vi "CANOpen_SDO Read RW.vi"(8 "error in":errorcluster, 11 "SDO Asynch in":T1 {"HW Dyn Read"."Resp Chan."."Chan Refs" format="%.0x"; "HW Dyn Read"."Req Chan."."Chan Refs" format="%.0x"; "HW Dyn Write"."Resp Chan."."Chan Refs" format="%.0x"; "HW Dyn Write"."Req Chan."."Chan Refs" format="%.0x"; "List SDO"."Resp Chan."."Chan Refs" format="%.0x"; "List SDO"."Req Chan."."Chan Refs" format="%.0x"}) -> (0 "error out":errorcluster, 3 "SDO Asynch out":T1 {"HW Dyn Read"."Resp Chan."."Chan Refs" format="%.0x"; "HW Dyn Read"."Req Chan."."Chan Refs" format="%.0x"; "HW Dyn Write"."Resp Chan."."Chan Refs" format="%.0x"; "HW Dyn Write"."Req Chan."."Chan Refs" format="%.0x"; "List SDO"."Resp Chan."."Chan Refs" format="%.0x"; "List SDO"."Req Chan."."Chan Refs" format="%.0x"})   [LabVIEW 2021, in "CANOpen Addon Engine.lvlib"]
uses:
  CANOpen Addon Engine.lvlib
  CANOpen_VS SDOs Data Refs.ctl
  <vilib>/NI VeriStand/Custom Device API/Data Reference.ctl
  Async VIs/CANOpen_Main/SubVIs/CanOpen_SDO Dynamic queue.ctl
  Shared/CANOpen_SDO queue W data.ctl
  Shared/CANOpen_SDO queue mode.ctl
  Shared/CANOpen_PDO Data Type in queue.ctl
  <vilib>/NI VeriStand/Custom Device API/Global Data Refs.vi
  <vilib>/NI VeriStand/Custom Device API/Custom Device API.lvlib
  Debug/SubVIs/Global debug.vi
  Shared/CANOpen Addon Shared.lvlib
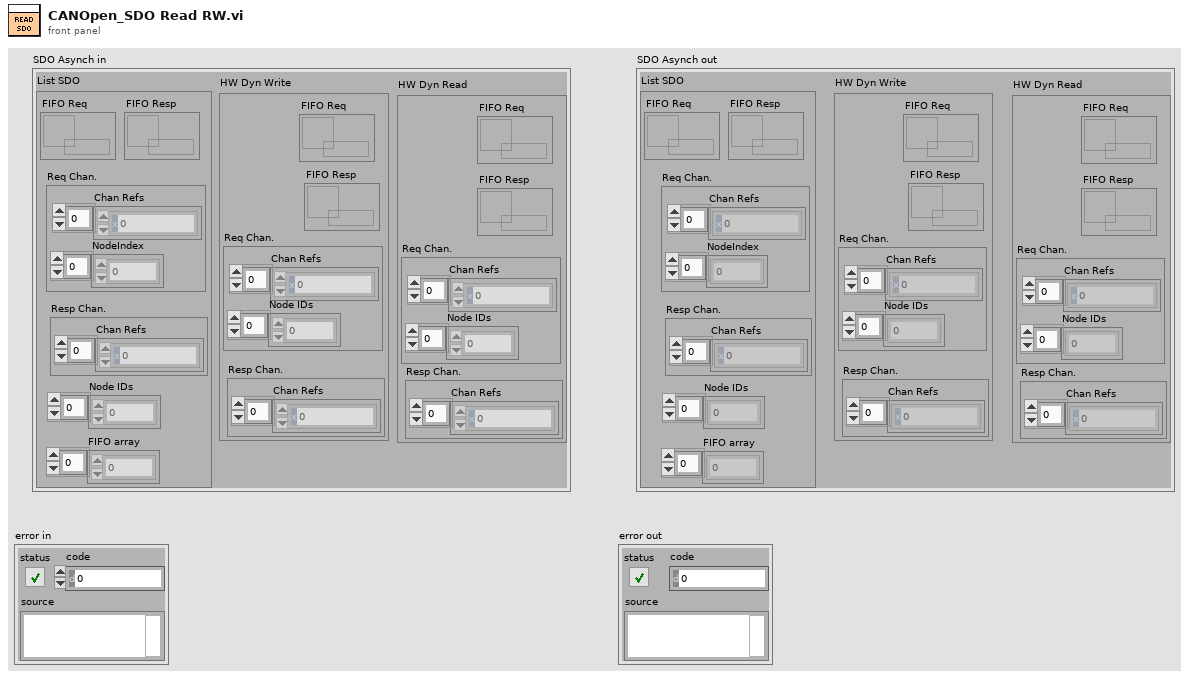
[diagram p1: front panel]
types:
  T1 = typedef "CANOpen Addon Engine.lvlib/CANOpen_VS SDOs Data Refs.ctl" = cluster{"List SDO":cluster{"FIFO Req":refnum<k33>, "Req Chan.":cluster{"Chan Refs":T2[], "NodeIndex":dbl[]}, "FIFO Resp":refnum<k33>, "Resp Chan.":cluster{"Chan Refs":T2[]}, "Node IDs":u8[], "FIFO array":dbl[]}, "HW Dyn Write":cluster{"FIFO Req":refnum<k33>, "FIFO Resp":refnum<k33>, "Req Chan.":cluster{"Chan Refs":T2[], "Node IDs":u8[]}, "Resp Chan.":cluster{"Chan Refs":T2[]}}, "HW Dyn Read":cluster{"FIFO Req":refnum<k33>, "FIFO Resp":refnum<k33>, "Req Chan.":cluster{"Chan Refs":T2[], "Node IDs":u8[]}, "Resp Chan.":cluster{"Chan Refs":T2[]}}}
  T2 = typedef "Custom Device API.lvlib/Data Reference.ctl" = i32
  T3 = typedef "CANOpen Addon Shared.lvlib/CANOpen_SDO queue mode.ctl" = enum16{"WRITE write", "WRITE response", "READ write", "READ response"}
  T4 = typedef "CANOpen Addon Engine.lvlib/CanOpen_SDO Dynamic queue.ctl" = cluster{"Node ID":u8, "Data":T5}
  T5 = typedef "CANOpen Addon Shared.lvlib/CANOpen_SDO queue W data.ctl" = cluster{"Object Index":u16, "Object Sub-Index (0)":u8, "Mode":T3, "Data Type":T6, "Value":dbl, "Status code":dbl, "Byte Order":enum16{"big-endian, network order", "little-endian"}}
  T6 = typedef "CANOpen Addon Shared.lvlib/CANOpen_PDO Data Type in queue.ctl" = enum16{"U8", "U16", "U32", "I8", "I16", "I32", "Single", "Double"}
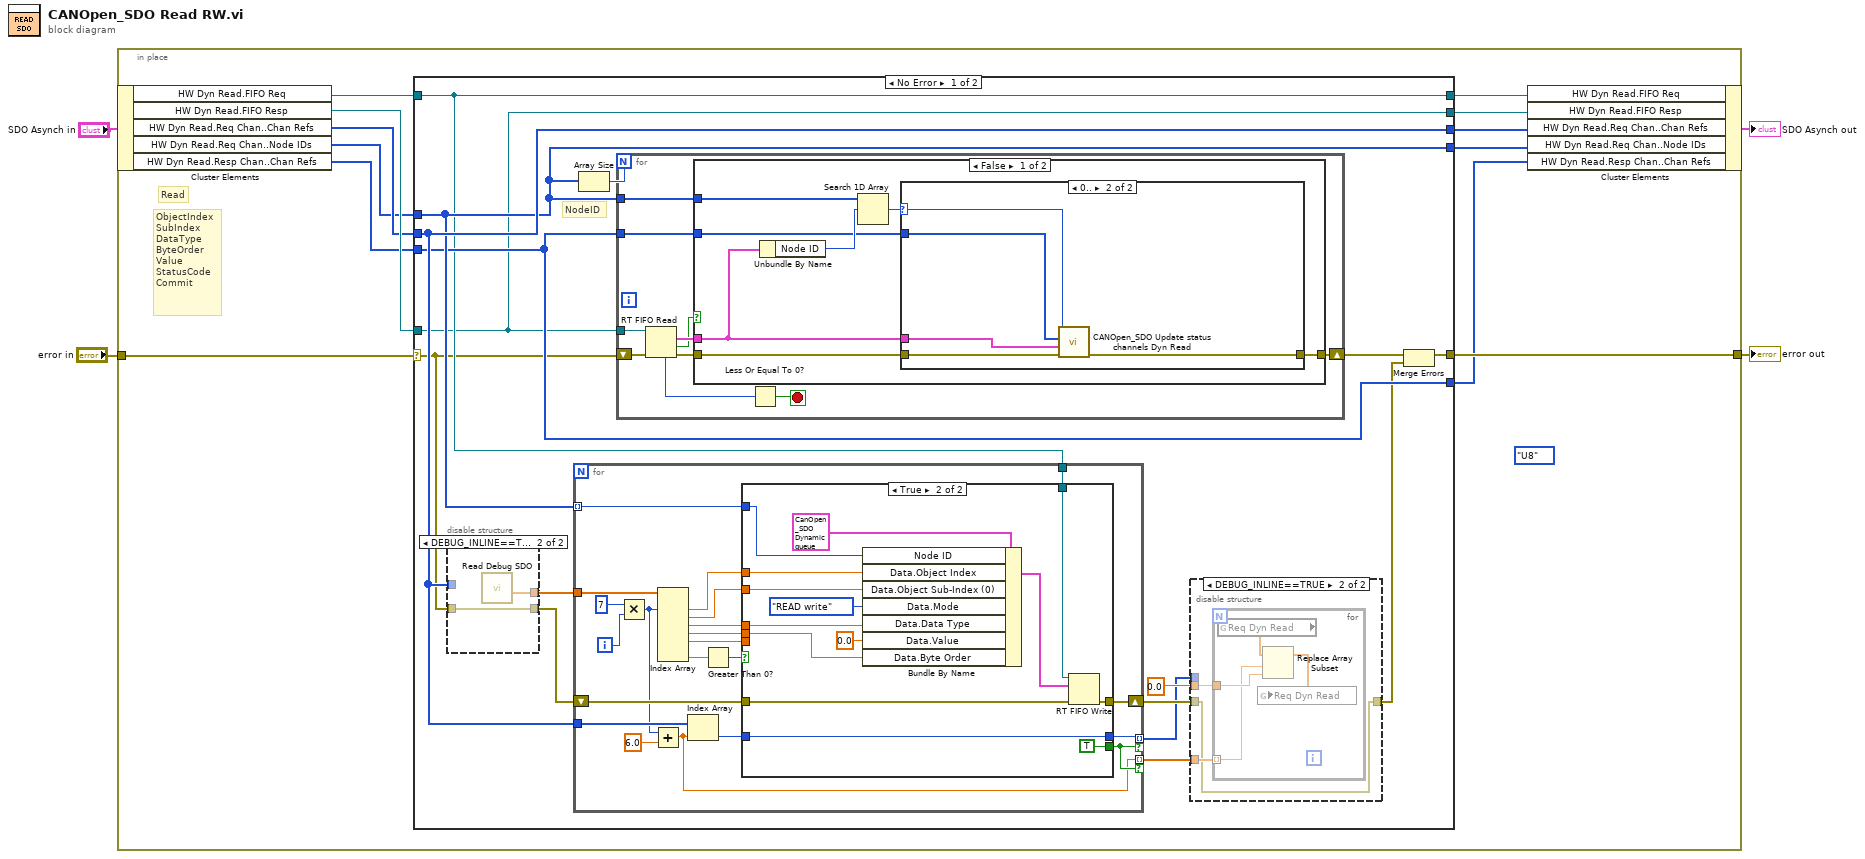
[diagram p0: block diagram]
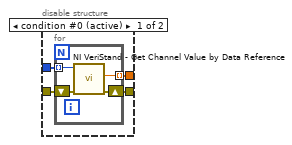
[diagram p4: hidden frame]
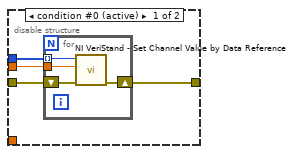
[diagram p5: hidden frame]
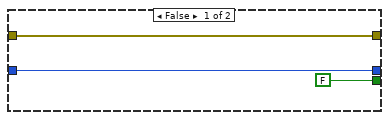
[diagram p6: hidden frame]
diagram:
  n1 = in-place {
    in-place-border: "error in" -> [w11]
    in-place-border: [w10] -> w1
    (unwired) CANOpen_PDO_Data_Type_in_queue."U8" ("Data.Data Type")
    # "Read"
    # "ObjectIndex\nSubIndex\nDataType\nByteOrder\nValue\nStatusCode\nCommit"
    n2 = in-place-cluster #1("SDO Asynch in") -> ("HW Dyn Read.FIFO Req"=w12:refnum<k33>, "HW Dyn Read.FIFO Resp"=w16:refnum<k33>, "HW Dyn Read.Req Chan..Chan Refs"=w14:T2[], "HW Dyn Read.Req Chan..Node IDs"=w5:u8[], "HW Dyn Read.Resp Chan..Chan Refs"=w9:T2[])
    n3 = case shown="No Error" w11 {
      selector: w11 -> [w17 w121]
      tunnel: [w28 w121] -> w10
      tunnel: w16 -> [w18 w125]
      tunnel: [w18 w125] -> w15
      tunnel: w14 -> [w31 w124]
      tunnel: w5 -> [w30 w123]
      tunnel: [w31 w124] -> w13
      tunnel: [w30 w123] -> w6
      tunnel: w12 -> [w21 w122]
      tunnel: w9 -> [w29 w120]
      tunnel: [w21 w122] -> w8
      tunnel: [w29 w120] -> w7
      frame No Error {
        # "NodeID"
        n4 = disable-structure shown="DEBUG_INLINE==TRUE" {
          disable-tunnel: w31 -> [w60 _]
          disable-tunnel: w17 -> [w59 w66]
          disable-tunnel: [w58 w66] -> w25
          disable-tunnel: [w57 w65] -> w26
          frame condition #0 (active) {
            n5 = for {
              tunnel: w60 -> [w64] mode=indexing
              tunnel: [w63] -> w57 mode=indexing
              shift-right: [w61] -> w58
              shift-left: w59 -> [w62]
              n6 = call <vilib>:"NI VeriStand - Get Channel Value by Data Reference.vi"("error in (no error)"=w62, "Data Reference in"=w64) -> ("error out"=w61:errorcluster, "Value"=w63:dbl)  [unwired: 8 in]
            }
          }
          frame condition #1 {
            n7 = call "Read Debug SDO.vi"() -> ("Req Dyn Read"=w65:dbl[])  [unwired: 8 in, 3 out]
          }
        }
        n8 = for {
          tunnel: w30 -> [w98] mode=indexing
          tunnel: w26 -> [w102]
          shift-right: [w92] -> w23
          shift-left: w25 -> [w93]
          tunnel: w31 -> [w91]
          tunnel: [w87] -> w22 mode=indexing if=w84
          tunnel: w21 -> [w86]
          tunnel: [w82] -> w20 mode=indexing if=w84
          i -> [w85]
          n9 = Multiply(x=7, y=w85) -> (x*y=w89:i32)
          n10 = Add(x=w89, y=6.0) -> (x+y=w82:dbl)
          n11 = Index Array(array=w102, index #1=w89) -> (element #1=w97:dbl, element #2=w96:dbl, element #3=w95:dbl, element #4=w94:dbl, element #5=w83:dbl, element #7=w100:dbl)  [unwired: 6 in, 1 out]
          n12 = Index Array(array=w91, index=w82) -> (element=w88:T2)
          n13 = Greater Than 0?(x=w100) -> (x > 0?=w99:bool)
          n14 = case shown="True" w99 {
            tunnel: [w105 w119] -> w92
            tunnel: w98 -> [_ w107]
            tunnel: w97 -> [_ w116]
            tunnel: w96 -> [_ w115]
            tunnel: w95 -> [_ w113]
            tunnel: w94 -> [_ w112]
            tunnel: w83 -> [_ _]
            tunnel: w93 -> [w105 w111]
            tunnel: w88 -> [w104 w109]
            tunnel: [w104 w109] -> w87
            tunnel: [FALSE TRUE] -> w84
            tunnel: w86 -> [_ w108]
            frame False {
            }
            frame True {
              n15 = Bundle By Name(cluster=T4 {"Node ID"=0, "Data"={"Object Index"=0, "Object Sub-Index (0)"=0, "Mode"=enum."WRITE write", "Data Type"=enum."U8", "Value"=0.0, "Status code"=0.0, "Byte Order"=enum."little-endian"}} ("element"), "Node ID"=w107, "Data.Object Index"=w116, "Data.Object Sub-Index (0)"=w115, "Data.Mode"=CANOpen_SDO_queue_mode."READ write", "Data.Data Type"=w113, "Data.Value"=0.0, "Data.Byte Order"=w112) -> (w117:T4)
              n16 = RT FIFO Write(0:w108, 1:w117, 3:w111) -> (11:w119:errorcluster)  [unwired: 2 in, 3 out]
            }
          }
        }
        n17 = Array Size(array=w30) -> (size(s)=w19:i32)
        n18 = for {
          N: w19 -> [_]
          tunnel: w30 -> [w38]
          tunnel: w18 -> [w40]
          shift-right: [w35] -> w32
          shift-left: w17 -> [w39]
          tunnel: w29 -> [w37]
          stop <- w41 stop-if-true
          n19 = RT FIFO Read(0:w40, 3:w39) -> (7:w42:u32, 9:w34:T4, 10:w33:bool, 11:w36:errorcluster)  [unwired: 2 in, 1 out]
          n20 = case shown="False" w33 {
            tunnel: w38 -> [w49 _]
            tunnel: w37 -> [w46 _]
            tunnel: w36 -> [w45 w56]
            tunnel: [w44 w56] -> w35
            tunnel: w34 -> [w43 _]
            frame False {
              n21 = Unbundle By Name(w43) -> ("Node ID"=w48:u8)
              n22 = Search 1D Array(1D array=w49, element=w48) -> (index of element=w47:i32)  [unwired: 1 in]
              n23 = case shown="0.." w47 {
                selector: w47 -> [_ w55]
                tunnel: w46 -> [_ w54]
                tunnel: w45 -> [w50 w53]
                tunnel: [w50 w52] -> w44
                tunnel: w43 -> [_ w51]
                frame -1, Default {
                }
                frame 0.. {
                  n24 = call "CANOpen_SDO Update status channels Dyn Read.vi"("error in (no error)"=w53, "Status Data"=w51, "Chan Refs"=w54, "index of element"=w55) -> ("error out"=w52:errorcluster)  [unwired: 7 in]
                }
              }
            }
            frame True {
            }
          }
          n25 = Less Or Equal To 0?(x=w42) -> (x <= 0?=w41:bool)
        }
        n26 = disable-structure shown="DEBUG_INLINE==TRUE" {
          disable-tunnel: [w70 w75] -> w27
          disable-tunnel: w23 -> [w69 w75]
          disable-tunnel: w22 -> [w68 _]
          disable-tunnel: 0.0 ("Value") -> [w67 w77]
          disable-tunnel: w20 -> [_ w76]
          frame condition #0 (active) {
            n27 = for {
              tunnel: w68 -> [w72] mode=indexing
              shift-right: [w73] -> w70
              shift-left: w69 -> [w74]
              tunnel: w67 -> [w71]
              n28 = call <vilib>:"NI VeriStand - Set Channel Value by Data Reference.vi"("error in (no error)"=w74, "Value"=w71, "Data Reference in"=w72) -> ("error out"=w73:errorcluster)  [unwired: 8 in]
            }
          }
          frame condition #1 {
            n29 = for {
              tunnel: w77 -> [w79]
              tunnel: w76 -> [w78] mode=indexing
              n30 = global read "Global debug.vi" "Req Dyn Read"() -> (w80:dbl[])
              n31 = Replace Array Subset(array=w80, new element=w79, index=w78) -> (w81:dbl[])
              n32 = global write "Global debug.vi" "Req Dyn Read"(w81) -> ()
            }
          }
        }
        n33 = Merge Errors(w32, w27) -> (w28:errorcluster)
      }
      frame Error {
      }
    }
    n34 = in-place-cluster #1("HW Dyn Read.FIFO Req"=w8, "HW Dyn Read.FIFO Resp"=w15, "HW Dyn Read.Req Chan..Chan Refs"=w13, "HW Dyn Read.Req Chan..Node IDs"=w6, "HW Dyn Read.Resp Chan..Chan Refs"=w7) -> (→"SDO Asynch out":T1)
  }
  "error out" <- w1
